vi "CRYAPI Set Active Window.vi"(10 "nData":i32) -> ()   [LabVIEW 2013]
uses:
  CRYMain Sub Window Global.vi
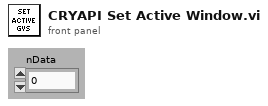
[diagram p1: front panel]
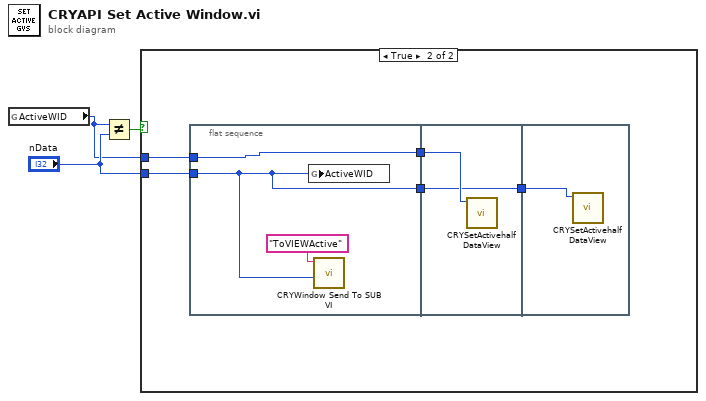
[diagram p0: block diagram]
diagram:
  n1 = global read "CRYMain Sub Window Global.vi" "ActiveWID"() -> (w1:i32)
  n2 = Not Equal?(x=w1, y="nData") -> (x != y?=w3:bool)
  n3 = case shown="True" w3 {
    tunnel: "nData" -> [_ w8]
    tunnel: w1 -> [_ w7]
    frame False {
    }
    frame True {
      n4 = flat-sequence {
        tunnel: w8 -> [w9]
        tunnel: w7 -> [w10]
        tunnel: [w10] -> w6
        tunnel: [w9] -> w4
        tunnel: w6 -> [w13]
        tunnel: [w12] -> w5
        tunnel: w4 -> [w12]
        tunnel: w5 -> [w14]
        frame #0 {
          n5 = global write "CRYMain Sub Window Global.vi" "ActiveWID"(w9) -> ()
          n6 = call "CRYWindow Send To SUB VI.vi"("nData"=w9, "sAction"="ToVIEWActive") -> ()  [unwired: 9 in, 1 out]
        }
        frame #1 {
          n7 = call "CRYSetActivehalf DataView.vi"("Frame nID"=w13) -> ()  [unwired: 11 in]
        }
        frame #2 {
          n8 = call "CRYSetActivehalf DataView.vi"("Frame nID"=w14) -> ()  [unwired: 11 in]
        }
      }
    }
  }
